vi "Query Voltage.vi"(8 "error in (no error)":errorcluster, 11 "E3631A in":refnum<class "E3631A.lvclass">) -> (0 "error out":errorcluster, 2 "Voltage":dbl, 3 "E3631A out":refnum<class "E3631A.lvclass">)   [LabVIEW 2020, in "E3631A.lvclass"]
uses:
  E3631A.lvclass
  C:/Sandbox/RF Bench/Source Code/WiSpry Test Framework/Instruments/Power Supply/Power Supply.lvclass
  C:/Sandbox/RF Bench/Source Code/WiSpry Test Framework/Instruments/Instrument.lvclass
  Instrument.lvclass/Instrument.ctl
  Power Supply.lvclass/Power Supply.ctl
  Instrument.lvclass
  Power Supply.lvclass
  <instrlib>/Agilent E363X Series/Agilent E363X Series.lvlib
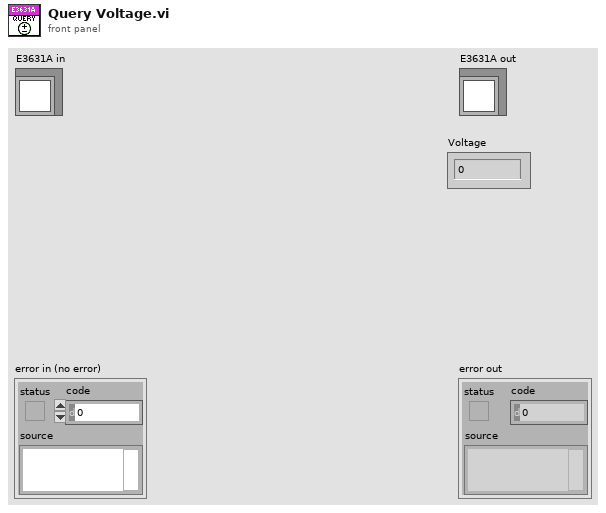
[diagram p1: front panel]
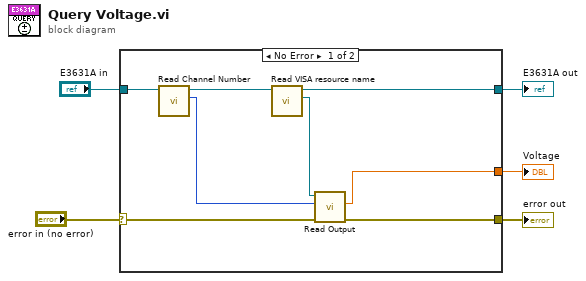
[diagram p0: block diagram]
diagram:
  n1 = case shown="No Error" "error in (no error)" {
    selector: "error in (no error)" -> [w8 w15]
    tunnel: [w7 w15] -> w5
    tunnel: "E3631A in" -> [w12 w14]
    tunnel: [w13 w14] -> w3
    tunnel: [w6 _] -> w4
    frame No Error {
      n2 = call "Read Channel Number.vi"("Power Supply in"=w12) -> ("Channel Number"=w9:u8, "Power Supply out"=w11:refnum<class "E3631A.lvclass">)  [unwired: 9 in]
      n3 = call "Read VISA resource name.vi"("Instrument in"=w11) -> ("VISA resource name"=w10:refnum<visa-resource-name>, "Instrument out"=w13:refnum<class "E3631A.lvclass">)  [unwired: 9 in]
      n4 = call <instrlib>:"Read Output.vi"("error in (no error)"=w8, "Channel (1: Channel 1)"=w9, "VISA resource name"=w10) -> ("error out"=w7:errorcluster, "Actual Voltage Level (V)"=w6:dbl)  [unwired: 5 in, 2 out]
    }
    frame Error {
    }
  }
  "error out" <- w5
  "E3631A out" <- w3
  "Voltage" <- w4
